vi "WinZip - Create Self-Extracting Archive.vi"(5 "AutoExtract w/o prompt? (F)":bool, 6 "Welcome Screen TXT file (none)":path, 7 "Title (none)":string, 8 "error in (no error)":errorcluster, 9 "Launch on Extract":path, 10 "Target Archive (.exe)":path, 11 "File or Folder Path":path) -> (0 "error out":errorcluster, 3 "Path to Archive":path)   [LabVIEW 2011]
uses:
  <userlib>/_OpenG.lib/file/file.llb/Convert File Extension (Path)__ogtk.vi
  <userlib>/_OpenG.lib/file/file.llb/File Exists - Scalar__ogtk.vi
  <userlib>/_OpenG.lib/file/file.llb/Append Path to Root if Relative - Scalar__ogtk.vi
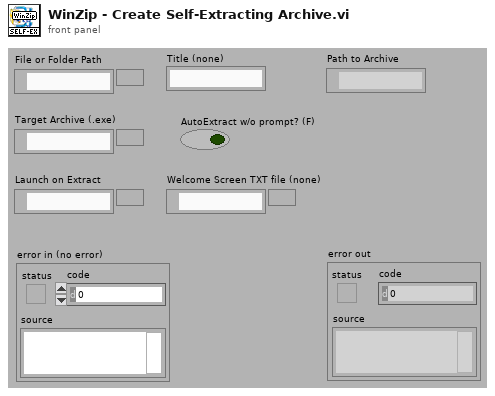
[diagram p1: front panel]
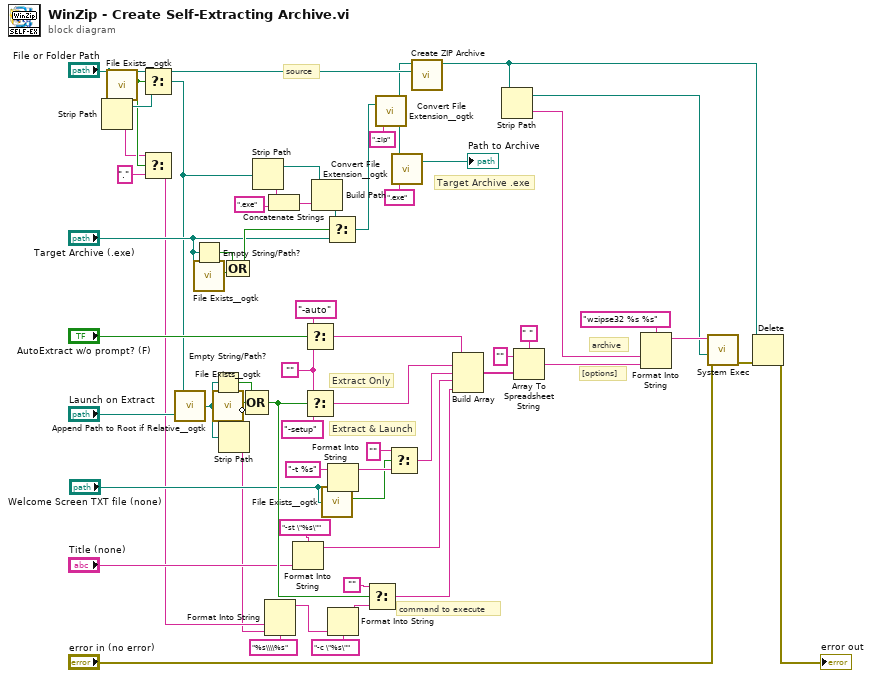
[diagram p0: block diagram]
diagram:
  w27 = ""
  # "archive"
  # "[options]"
  # "source"
  # "command to execute"
  # "Extract & Launch"
  # "Extract Only"
  # "Target Archive .exe"
  n1 = Strip Path(path="File or Folder Path") -> (stripped path=w60:path, name=w6:string)
  n2 = call-poly <userlib>:"File Exists__ogtk.vi"("file path"="File or Folder Path") -> ("is directory"=w7:bool)  [unwired: 6 in, 1 out]
  n3 = Select(t="File or Folder Path", s=w7, f=w60) -> (s? t:f=w26:path)
  n4 = Select(t=w6, s=w7, f=".") -> (s? t:f=w4:string)
  n5 = call-poly <userlib>:"Append Path to Root if Relative__ogtk.vi"("Absolute or Relative Path"="Launch on Extract", "Root Path"=w26) -> ("Absolute or Appended Path"=w41:path)
  n6 = Empty String/Path?(string/path="Target Archive (.exe)") -> (empty?=w53:bool)
  n7 = call-poly <userlib>:"File Exists__ogtk.vi"("file path"="Target Archive (.exe)") -> ("is directory"=w54:bool)  [unwired: 6 in, 1 out]
  n8 = Empty String/Path?(string/path=w41) -> (empty?=w59:bool)
  n9 = call-poly <userlib>:"File Exists__ogtk.vi"("file path"=w41) -> ("is directory"=w58:bool, "exists"=w57:bool)  [unwired: 6 in]
  n10 = Strip Path(path=w41) -> (name=w3:string)  [unwired: 1 out]
  n11 = Compound Arithmetic op=OR(w53, w54) -> (w48:bool)
  n12 = Compound Arithmetic op=OR(w59, w58, invert w57) -> (w55:bool)
  n13 = Strip Path(path=w26) -> (stripped path=w42:path, name=w52:string)
  n14 = Format Into String(format string="%s\\\\%s", w4, w3) -> (resulting string=w2:string)  [unwired: 2 in, 1 out]
  n15 = Concatenate Strings(w52, ".exe") -> (w50:string)
  n16 = Format Into String(format string="-st \"%s\"", "Title (none)") -> (resulting string=w16:string)  [unwired: 2 in, 1 out]
  n17 = Select(t="-auto", s="AutoExtract w/o prompt? (F)", f=w27) -> (s? t:f=w19:string)
  n18 = Select(t=w27, s=w55, f="-setup") -> (s? t:f=w18:string)
  n19 = Build Path(base path=w42, name or relative path=w50) -> (appended path=w49:path)
  n20 = call-poly <userlib>:"File Exists__ogtk.vi"("file path"="Welcome Screen TXT file (none)") -> ("is directory"=w34:bool)  [unwired: 6 in, 1 out]
  n21 = Select(t=w49, s=w48, f="Target Archive (.exe)") -> (s? t:f=w29:path)
  n22 = Format Into String(format string="-t %s", "Welcome Screen TXT file (none)") -> (resulting string=w35:string)  [unwired: 2 in, 1 out]
  n23 = Format Into String(format string="-c \"%s\"", w2) -> (resulting string=w31:string)  [unwired: 2 in, 1 out]
  n24 = Select(t="", s=w55, f=w31) -> (s? t:f=w15:string)
  n25 = call-poly <userlib>:"Convert File Extension__ogtk.vi"("new ending (none)"=".zip", "file name"=w29) -> ("new filename"=w25:path)  [unwired: 1 out]
  n26 = Select(t="", s=w34, f=w35) -> (s? t:f=w17:string)
  n27 = call-poly <userlib>:"Convert File Extension__ogtk.vi"("new ending (none)"=".exe", "file name"=w25) -> ("new filename"=→"Path to Archive":path)  [unwired: 1 out]
  n28 = call "Create ZIP Archive.vi"("Source File/Directory"="File or Folder Path", "Target Zip File"=w25) -> ("Path to .zip"=w9:path)  [unwired: 9 out]
  n29 = Build Array(w19, w18, w17, w16, w15) -> (w14:string[])
  n30 = Strip Path(path=w9) -> (stripped path=w8:path, name=w10:string)
  n31 = Array To Spreadsheet String(delimiter (Tab)=" ", array=w14, 3:"") -> (spreadsheet string=w11:string)
  n32 = Format Into String(format string="wzipse32 %s %s" ("command line"), w10, w11) -> (resulting string=w45:string)  [unwired: 2 in, 1 out]
  n33 = call <vilib>:"System Exec.vi"("error in (no error)"="error in (no error)", "working directory"=w8, "command line"=w45) -> ("error out"=w44:errorcluster)  [unwired: 3 in, 5 out]
  n34 = Delete(path (use dialog)=w9, error in=w44) -> (error out=→"error out":errorcluster)  [unwired: 5 out]
